vi "Thermocouples.vi"() -> ()   [LabVIEW 2017]
uses:
  <vilib>/Platform/TimedLoop/XDataNode/wakeup.ctl
  <vilib>/Platform/TimedLoop/XDataNode/XDNodeRunTimeDep.lvlib
  <vilib>/Platform/TimedLoop/XDataNode/nitl_modes.ctl
  <vilib>/Platform/TimedLoop/XDataNode/timing_clust.ctl
  <vilib>/platform/TimedLoop/XDataNode/XDataNode.xnode
  <vilib>/ptbypt/NI_PtbyPt.lvlib
  <vilib>/Platform/TimedLoop/XDataNode/loadnilvce.vi
panel:
  out "Numeric 4":dbl
  out "Numeric 3":dbl
  out "Numeric 2":dbl
  out "Numeric":dbl
  in  "stop":bool
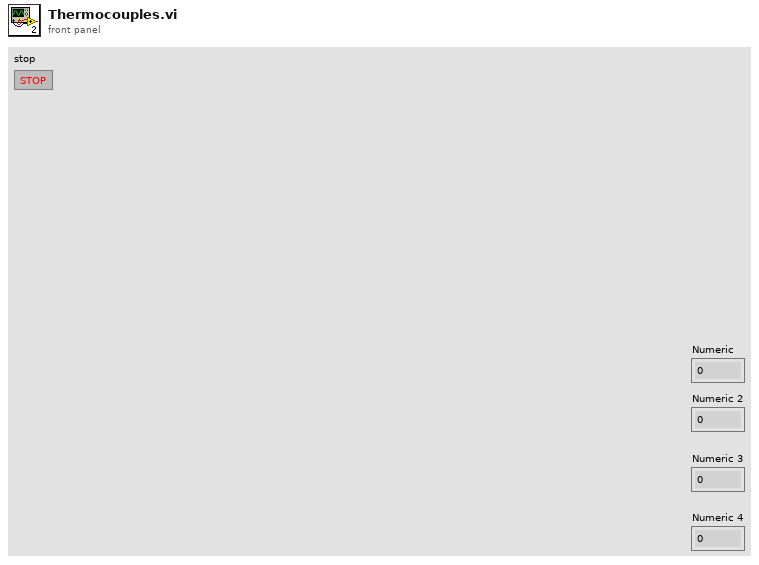
[diagram p1: front panel]
types:
  T1 = typedef "XDNodeRunTimeDep.lvlib/timing_clust.ctl" = cluster{"Expected End [f-1]":u64, "Actual End [f-1]":u64, "Finished Late? [f-1]":bool, "Expected End [i-1]":u64, "Actual End [i-1]":u64, "Finished Late? [i-1]":bool, "Expected Start [i]":u64, "Actual Start [i]":u64, "Expected Start [f]":u64, "Actual Start [f]":u64, "Source Name":string, "Structure Name":string, "Period":i64, "Deadline":i64, "Offset":i64, "Start":i64, "Priority":i32, "Timeout":i32, "Mode":T2, "Wakeup Reason":T3, "Error":errorcluster, "Source Type":string, "Secondary Source Type":string, "Global End Time":u64, "Global Start Time":u64, "Frame Duration":u64, "Iteration Duration":u64, "Assigned CPU":i32, "I/O Scan Engine Mode":u32}
  T2 = typedef "XDNodeRunTimeDep.lvlib/nitl_modes.ctl" = enum32{"No Change", "Process missed periods, maintain original phase", "Discard missed periods, maintain original phase", "Process missed periods, ignore original phase", "Discard missed periods, ignore original phase"}
  T3 = typedef "XDNodeRunTimeDep.lvlib/wakeup.ctl" = enum32{"Normal", "Aborted", "Asynchronous wakeup", "Timing source error", "Timed loop error", "Timeout"}
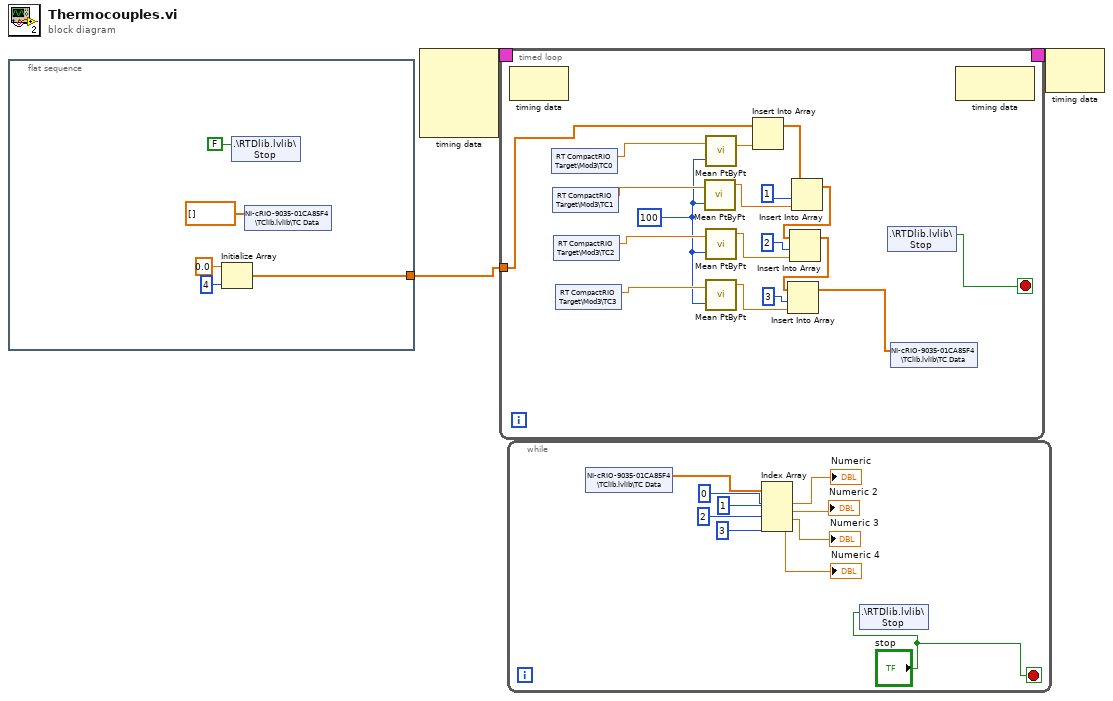
[diagram p0: block diagram]
diagram:
  n1 = flat-sequence {
    tunnel: [w5] -> w1
    frame #0 {
      n2 = Initialize Array(0.0 ("element"), 4 ("dimension size")) -> (w5:dbl[])
      n3 = shared-variable ".\\RTDlib.lvlib\\Stop"(FALSE ("Stop")) -> ()  [unwired: 1 in, 1 out]
      n4 = shared-variable "NI-cRIO-9035-01CA85F4\\TClib.lvlib\\TC Data"(dbl[] [] ("TC Data")) -> ()  [unwired: 1 in, 1 out]
    }
  }
  n5 = node-c288() -> (w3:T1)  [unwired: 4 in]
  n6 = timed-loop {
    timing: w3 -> [_]
    timing-out: [_] -> w2
    tunnel: w1 -> [w26]
    stop <- w21 stop-if-true
    w16 = 100
    n7 = node-c288() -> ()  [unwired: 1 in, 1 out]
    n8 = shared-variable "RT CompactRIO Target\\Mod3\\TC0"() -> (w20:dbl)  [unwired: 1 in, 1 out]
    n9 = shared-variable "RT CompactRIO Target\\Mod3\\TC1"() -> (w19:dbl)  [unwired: 1 in, 1 out]
    n10 = shared-variable "RT CompactRIO Target\\Mod3\\TC2"() -> (w18:dbl)  [unwired: 1 in, 1 out]
    n11 = shared-variable "RT CompactRIO Target\\Mod3\\TC3"() -> (w17:dbl)  [unwired: 1 in, 1 out]
    n12 = call <vilib>:"Mean PtByPt.vi"("x"=w19, "sample length"=w16) -> ("mean"=w23:dbl)  [unwired: 2 in, 1 out]
    n13 = call <vilib>:"Mean PtByPt.vi"("x"=w20, "sample length"=w16) -> ("mean"=w24:dbl)  [unwired: 2 in, 1 out]
    n14 = call <vilib>:"Mean PtByPt.vi"("x"=w18, "sample length"=w16) -> ("mean"=w11:dbl)  [unwired: 2 in, 1 out]
    n15 = call <vilib>:"Mean PtByPt.vi"("x"=w17, "sample length"=w16) -> ("mean"=w15:dbl)  [unwired: 2 in, 1 out]
    n16 = Insert Into Array(array=w26, new element=w24) -> (w25:dbl[])  [unwired: 1 in]
    n17 = Insert Into Array(array=w25, index=1, new element=w23) -> (w14:dbl[])
    n18 = Insert Into Array(array=w14, index=2, new element=w11) -> (w13:dbl[])
    n19 = Insert Into Array(array=w13, index=3, new element=w15) -> (w9:dbl[])
    n20 = shared-variable ".\\RTDlib.lvlib\\Stop"() -> (w21:bool)  [unwired: 1 in, 1 out]
    n21 = shared-variable "NI-cRIO-9035-01CA85F4\\TClib.lvlib\\TC Data"(w9) -> ()  [unwired: 1 in, 1 out]
    n22 = node-c288() -> ()  [unwired: 1 in, 1 out]
  }
  n23 = while {
    stop <- "stop" stop-if-true
    n24 = shared-variable "NI-cRIO-9035-01CA85F4\\TClib.lvlib\\TC Data"() -> (w37:dbl[])  [unwired: 1 in, 1 out]
    n25 = Index Array(array=w37, index #1=0 ("index"), index #2=1 ("index"), index #3=2 ("index"), index #4=3 ("index")) -> (element #1=→"Numeric":dbl, element #2=→"Numeric 2":dbl, element #3=→"Numeric 3":dbl, element #4=→"Numeric 4":dbl)
    n26 = shared-variable ".\\RTDlib.lvlib\\Stop"("stop") -> ()  [unwired: 1 in, 1 out]
  }
  n27 = node-c288(w2) -> ()  [unwired: 1 out]
